vi "escape.vi"(7 "Type":u16(ring) items=["escape", "Unescape"], 11 "Input String":string) -> (3 "Output string":string)   [LabVIEW 2020, in "MSXML.lvlib"]
uses:
  MSXML.lvlib
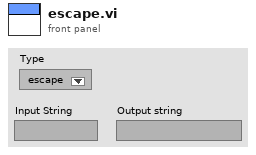
[diagram p1: front panel]
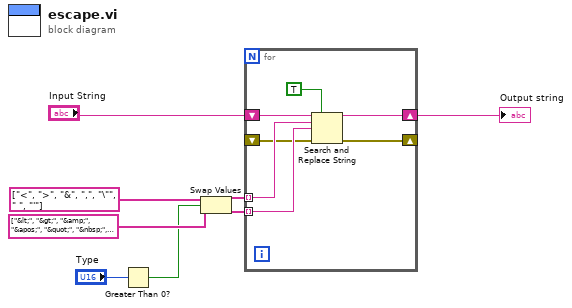
[diagram p0: block diagram]
diagram:
  n1 = Greater Than 0?(x="Type") -> (x > 0?=w2:bool)
  n2 = Swap Values(12:string[] ["<", ">", "&", ",", "\"", " ", "'"] ("search string"), 13:w2, 14:string[] ["&lt;", "&gt;", "&amp;", "&apos;", "&quot;", "&nbsp;", "&apos"] ("search string")) -> (1:w4:string[], 3:w5:string[])
  n3 = for {
    tunnel: w4 -> [w14] mode=indexing
    tunnel: w5 -> [w13] mode=indexing
    shift-right: [w12] -> w1
    shift-left: "Input String" -> [w15]
    shift-right: [w10] -> _
    shift-left: _ -> [w9]
    n4 = Search and Replace String(replace all?=TRUE ("replace all? (F)"), input string=w15, search string=w14, replace string=w13, error in=w9) -> (result string=w12:string, error out=w10:errorcluster)  [unwired: 3 in, 2 out]
  }
  "Output string" <- w1
